vi "AP2_doubling_spline_generation.vi"() -> ()   [LabVIEW 2023]
panel:
  in  "Main Control Tab":enum32{"Controls", "Monitoring"}(tab)
  in  "stop":bool
  in  "Step Size / nm":dbl
  in  "Lower Bound / nm":dbl
  in  "Upper bound / nm":dbl
  in  "Start Optimisation":bool
  in  "Cancel Optimisation":bool
  in  "BBO Motor Step Size":i32
  in  "BBO Start Position":i32
  in  "Initial Step Direction":u16
  in  "Averaging Time / s":u32
  out "RT Laser Power / J":dbl
  out "XY Graph":cluster{dbl[], dbl[]}(graph)
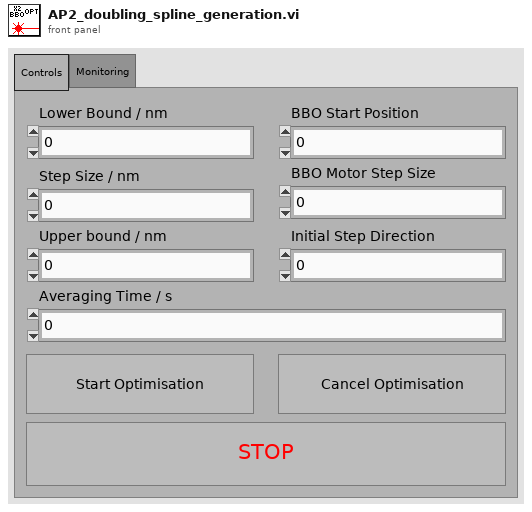
[diagram p1: front panel]
types:
  T1 = cluster{"queue out":refnum<queue>, "error out":errorcluster}
  T2 = cluster{"OphirLMMeasurementLib.ICoLMMeasurement2":refnum<k7>, "Error":errorcluster, "hDevice":i32}
  T3 = cluster{"BBO Start Position":i32, "Step Size":i32, "Initial Step Direction":u16, "Averaging Time / s ":u32}
  T4 = cluster{"Upper bound":dbl, "Step Size":dbl, "Lower Bound":dbl}
  T5 = cluster{"Power Reading ":dbl, "T imestamp":dbl, "Status":i32}
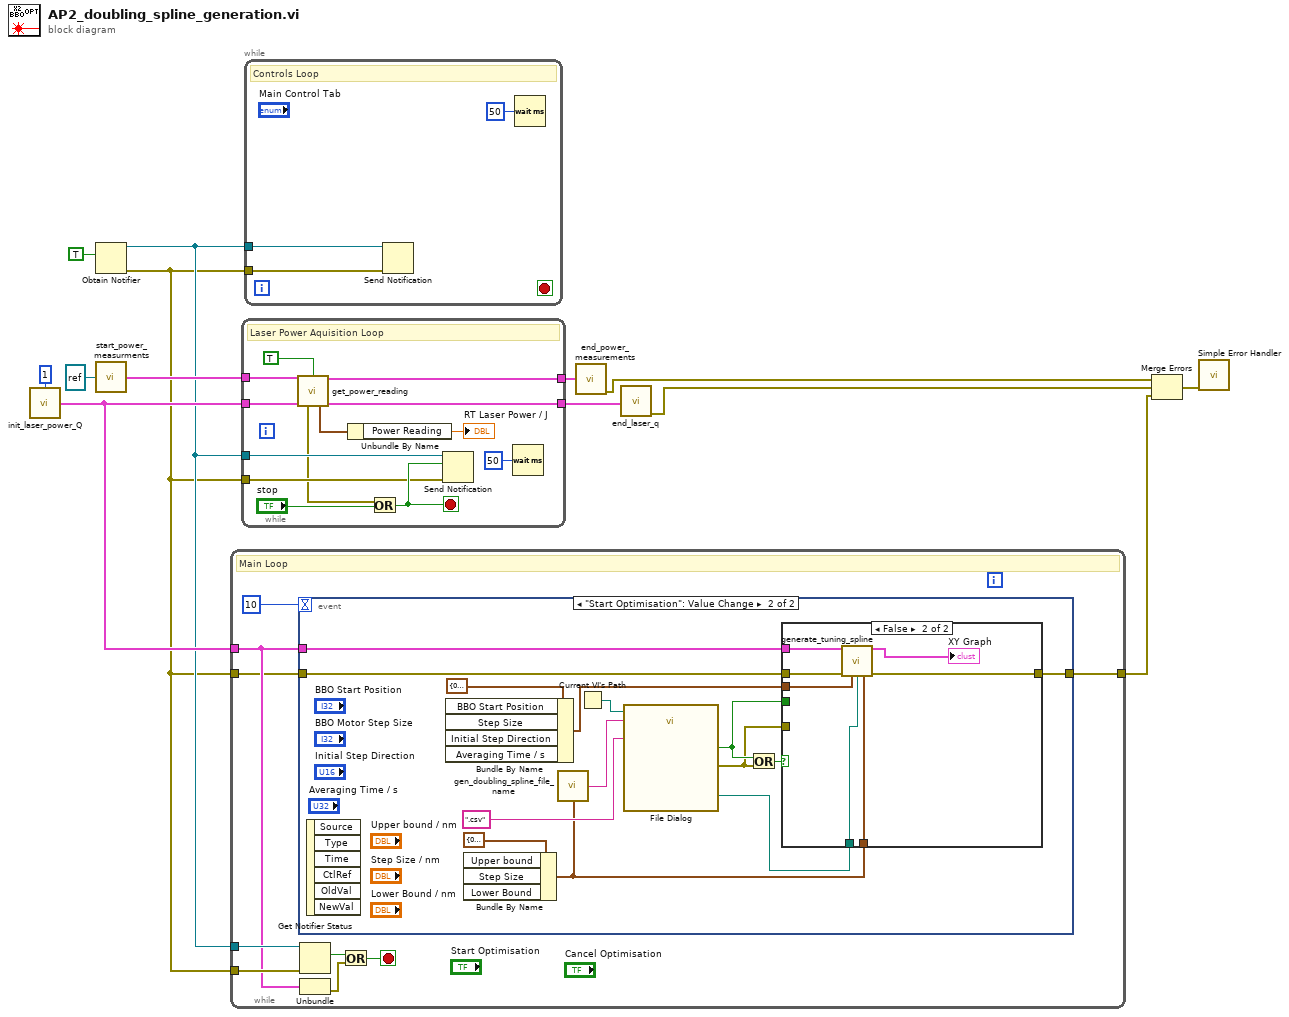
[diagram p0: block diagram]
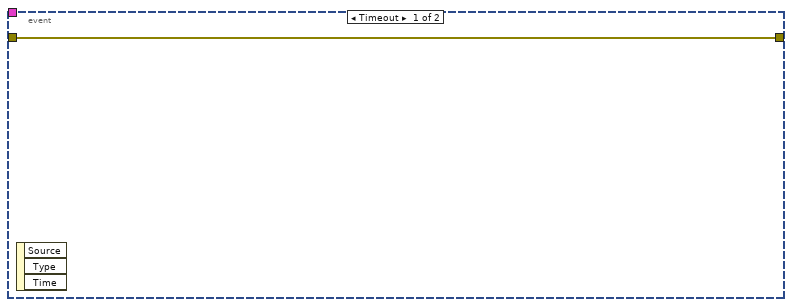
[diagram p2: hidden frame]
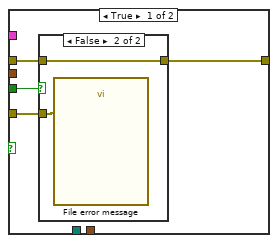
[diagram p3: hidden frame]
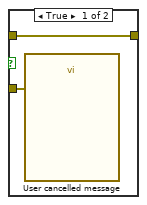
[diagram p4: hidden frame]
diagram:
  n1 = call "init_laser_power_Q.vi"("max queue size (-1, unlimited)"=1) -> ("Laser Power Q"=w4:T1)  [unwired: 14 in]
  n2 = Obtain Notifier(notification data type=TRUE) -> (notifier out=w2:refnum<notifier>, error out=w1:errorcluster)  [unwired: 3 in, 1 out]
  n3 = call "start_power_measurments.vi"("OphirLMMeasurementLib.ICoLMMeasurement2"=refnum<k7> refnum) -> ("Power Meter Connection Data Out"=w13:T2)  [unwired: 14 in]
  n4 = while {
    tunnel: w4 -> [w16]
    tunnel: w2 -> [w21]
    tunnel: w1 -> [w20]
    tunnel: w1 -> [w15]
    tunnel: [w14] -> w3
    stop <- w19 stop-if-true
    # "Main Loop"
    n5 = event shown="[1] \"Start Optimisation\": Value Change" {
      selector: _ -> [_ _]
      dyn-events: _ -> [_ _]
      timeout: 10 -> [_ _]
      tunnel: w16 -> [_ w36]
      tunnel: w15 -> [w23 w35]
      tunnel: [w23 w34] -> w14
      event Timeout {
        n6 = event-data() -> ()  [unwired: 1 in, 3 out]
      }
      event "Start Optimisation": Value Change {
        n7 = event-data() -> ()  [unwired: 1 in, 6 out]
        n8 = Bundle By Name(cluster=T3 {"BBO Start Position"=0, "Step Size"=0, "Initial Step Direction"=0, "Averaging Time / s "=0} ("Controls Cluster")) -> (w32:T3)  [unwired: 4 in]
        n9 = Bundle By Name(cluster=T4 {"Upper bound"=0.0, "Step Size"=0.0, "Lower Bound"=0.0}) -> (w24:T4)  [unwired: 3 in]
        n10 = call "gen_doubling_spline_file_name.vi"("output cluster"=w24) -> ("concatenated string"=w25:string)  [unwired: 14 in]
        n11 = Current VI's Path() -> (path=w27:path)
        n12 = call "File Dialog"("start path"=w27, "default name"=w25, "pattern (all files)"=".csv" ("pattern label")) -> ("selected path"=w30:path, "cancelled"=w29:bool, "error out"=w28:errorcluster)  [unwired: 9 in, 1 out]
        n13 = Or(x=w29, y=w28) -> (x .or. y?=w31:bool)
        n14 = case shown="False" w31 {
          tunnel: w36 -> [_ w52]
          tunnel: w24 -> [_ w48]
          tunnel: w35 -> [w41 w51]
          tunnel: [w40 w50] -> w34
          tunnel: w32 -> [_ w49]
          tunnel: w30 -> [_ w47]
          tunnel: w29 -> [w39 _]
          tunnel: w28 -> [w38 _]
          frame True {
            n15 = case shown="False" w39 {
              tunnel: w41 -> [w42 w44]
              tunnel: [w42 w44] -> w40
              tunnel: w38 -> [w43 w45]
              frame True {
                n16 = call "User cancelled message"("error in (no error)"=w43) -> ()  [unwired: 9 in, 2 out]
              }
              frame False {
                n17 = call "File error message"("error in (no error)"=w45) -> ()  [unwired: 9 in, 2 out]
              }
            }
          }
          frame False {
            n18 = call "generate_tuning_spline.vi"("Laser Power Q"=w52, "error in"=w51, "Controls Cluster"=w49, "file path (dialog if empty)"=w47, "Bounds"=w48) -> ("Opt Data"=→"XY Graph":cluster{dbl[], dbl[]}, "error out"=w50:errorcluster)  [unwired: 9 in]
          }
        }
      }
    }
    n19 = Get Notifier Status(notifier=w21, error in (no error)=w20) -> (current notification=w18:bool)  [unwired: 4 out]
    n20 = Unbundle(w16) -> ("error out"=w17:errorcluster)  [unwired: 1 out]
    n21 = Or(x=w18, y=w17) -> (x .or. y?=w19:bool)
  }
  n22 = while {
    tunnel: w13 -> [w64]
    tunnel: w4 -> [w63]
    tunnel: [w62] -> w11
    tunnel: [w61] -> w10
    tunnel: w2 -> [w58]
    tunnel: w1 -> [w57]
    stop <- w59 stop-if-true
    # "Laser Power Aquisition Loop"
    n23 = call "get_power_reading.vi"("Power Meter Connection Data In"=w64, "Q Laser Data?"=TRUE, "Laser Power Q In"=w63) -> ("Power Meter Connection Data Out"=w62:T2, "error out"=w54:errorcluster, "Data Out"=w55:T5, "Laser Power Q Out"=w61:T1)  [unwired: 9 in]
    n24 = Unbundle By Name(w55) -> ("Power Reading"=→"RT Laser Power / J":dbl)
    n25 = Or(x=w54, y="stop") -> (x .or. y?=w59:bool)
    n26 = Send Notification(notification=w59, notifier=w58, error in (no error)=w57) -> ()  [unwired: 2 out]
    n27 = Wait (ms)(milliseconds to wait=u32 50) -> ()  [unwired: 1 out]
  }
  n28 = while {
    tunnel: w2 -> [w67]
    tunnel: w1 -> [w66]
    stop <- _ stop-if-true
    # "Controls Loop"
    n29 = Send Notification(notifier=w67, error in (no error)=w66) -> ()  [unwired: 1 in, 2 out]
    n30 = Wait (ms)(milliseconds to wait=u32 50) -> ()  [unwired: 1 out]
  }
  n31 = call "end_power_measurements.vi"("Power Meter Connection Data In"=w11) -> ("error out"=w7:errorcluster)  [unwired: 14 in]
  n32 = call "end_laser_q.vi"("Laser Power Q In"=w10) -> ("error out"=w6:errorcluster)  [unwired: 14 in]
  n33 = Merge Errors(w7, w6, w3) -> (w5:errorcluster)
  n34 = call <vilib>:"Simple Error Handler.vi"("error in (no error)"=w5) -> ()  [unwired: 4 in, 5 out]
